vi "Edit Popup Menu.vi"(6 "User Menu States":bool[](array[boolean]), 7 "User Menu Items":string[](array[string]), 8 "error in (no error)":errorcluster, 10 "Menu Operation Cluster":T1(array[cluster]), 11 "Menu Ref In":refnum<k9>) -> (0 "error out":errorcluster, 3 "Menu Ref Out":refnum<k9>)   [LabVIEW 2017, in "2D Plot.lvclass"]
uses:
  <vilib>/Math Plots/2D Math Plots/2D Plot/2D Plot/2D Plot.lvclass
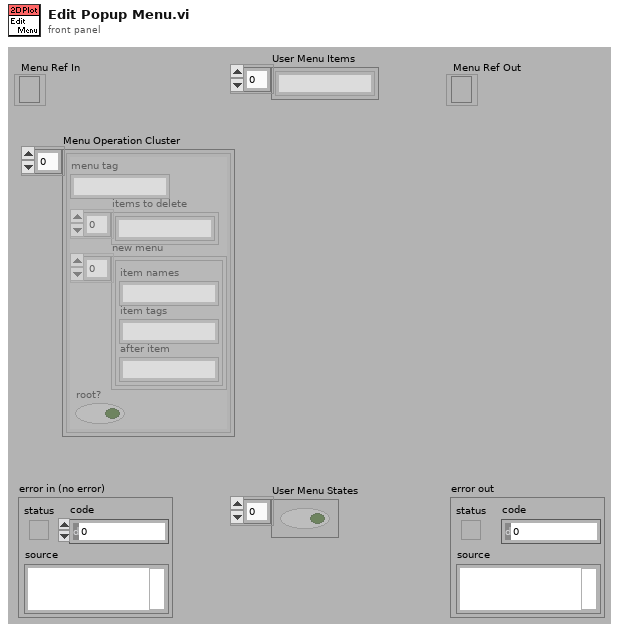
[diagram p1: front panel]
types:
  T1 = cluster{"menu tag":string, "items to delete":string[], "new menu":cluster{"item names":string, "item tags":string, "after item":string}[], "root?":bool}[]
  T2 = cluster{"item names":string, "item tags":string, "after item":string}[]
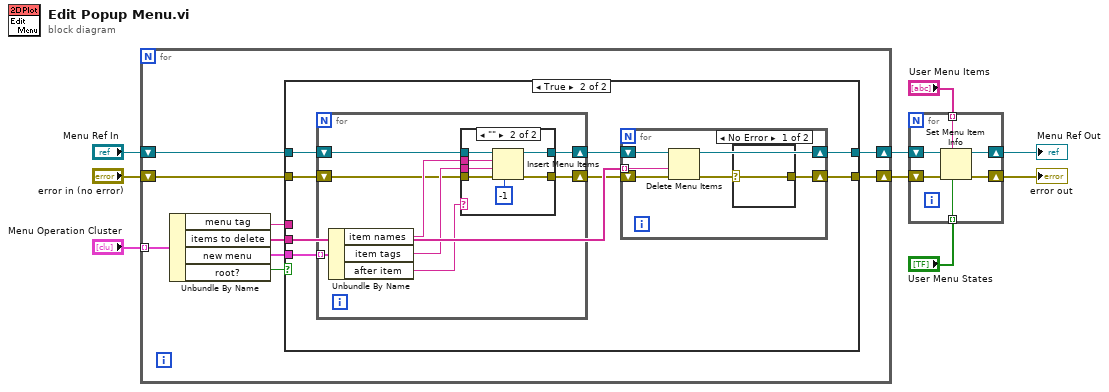
[diagram p0: block diagram]
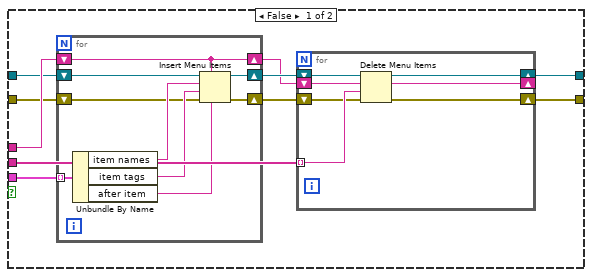
[diagram p2: hidden frame]
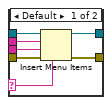
[diagram p3: hidden frame]
diagram:
  n1 = for {
    tunnel: "Menu Operation Cluster" -> [w18] mode=indexing
    shift-right: [w15] -> w6
    shift-left: "Menu Ref In" -> [w16]
    shift-right: [w11] -> w5
    shift-left: "error in (no error)" -> [w10]
    n2 = Unbundle By Name(w18) -> ("menu tag"=w14:string, "items to delete"=w13:string[], "new menu"=w12:T2, "root?"=w17:bool)
    n3 = case shown="True" w17 {
      tunnel: w16 -> [w20 w49]
      tunnel: w14 -> [w26 _]
      tunnel: w13 -> [w28 w50]
      tunnel: w12 -> [w27 w51]
      tunnel: [w21 w45] -> w15
      tunnel: [w22 w44] -> w11
      tunnel: w10 -> [w19 w48]
      frame False {
        n4 = for {
          shift-right: [w31] -> w24
          shift-left: w20 -> [w37]
          shift-right: [w36] -> w23
          shift-left: w26 -> [w36]
          tunnel: w27 -> [w35] mode=indexing
          shift-right: [w30] -> w25
          shift-left: w19 -> [w29]
          n5 = Unbundle By Name(w35) -> ("item names"=w34:string, "item tags"=w33:string, "after item"=w32:string)
          n6 = Insert Menu Items(4:w32, 5:w36, 6:w29, 7:w33, 8:w34, 9:w37) -> (0:w30:errorcluster, 3:w31:refnum<k9>)  [unwired: 1 out]
        }
        n7 = for {
          shift-right: [w42] -> w21
          shift-left: w24 -> [w43]
          shift-right: [w40] -> _
          shift-left: w23 -> [w40]
          tunnel: w28 -> [w41] mode=indexing
          shift-right: [w39] -> w22
          shift-left: w25 -> [w38]
          n8 = Delete Menu Items(6:w38, 7:w41, 8:w40, 9:w43) -> (0:w39:errorcluster, 3:w42:refnum<k9>)
        }
      }
      frame True {
        n9 = for {
          shift-right: [w59] -> w46
          shift-left: w49 -> [w58]
          tunnel: w51 -> [w57] mode=indexing
          shift-right: [w52] -> w47
          shift-left: w48 -> [w53]
          n10 = Unbundle By Name(w57) -> ("item names"=w56:string, "item tags"=w55:string, "after item"=w54:string)
          n11 = case shown="\"\"" w54 {
            selector: w54 -> [w64 _]
            tunnel: [w65 w73] -> w59
            tunnel: w58 -> [w66 w72]
            tunnel: w56 -> [w63 w71]
            tunnel: w55 -> [w62 w70]
            tunnel: w53 -> [w61 w68]
            tunnel: [w60 w67] -> w52
            frame Default {
              n12 = Insert Menu Items(4:w64, 6:w61, 7:w62, 8:w63, 9:w66) -> (0:w60:errorcluster, 3:w65:refnum<k9>)  [unwired: 2 out]
            }
            frame "" {
              n13 = Insert Menu Items(4:-1, 6:w68, 7:w70, 8:w71, 9:w72) -> (0:w67:errorcluster, 3:w73:refnum<k9>)  [unwired: 2 out]
            }
          }
        }
        n14 = for {
          shift-right: [w78] -> w45
          shift-left: w46 -> [w79]
          tunnel: w50 -> [w77] mode=indexing
          shift-right: [w74] -> w44
          shift-left: w47 -> [w76]
          n15 = Delete Menu Items(6:w76, 7:w77, 9:w79) -> (0:w75:errorcluster, 3:w78:refnum<k9>)  [unwired: 1 out]
          n16 = case shown="No Error" w75 {
            selector: w75 -> [w80 _]
            tunnel: [w80 _] -> w74
            frame No Error {
            }
            frame Error {
            }
          }
        }
      }
    }
  }
  n17 = for {
    shift-right: [w85] -> w1
    shift-left: w6 -> [w86]
    tunnel: "User Menu Items" -> [w84] mode=indexing
    tunnel: "User Menu States" -> [w83] mode=indexing
    shift-right: [w81] -> w9
    shift-left: w5 -> [w82]
    n18 = Set Menu Item Info(6:w83, 7:w84, 8:w82, 11:w86) -> (0:w81:errorcluster, 3:w85:refnum<k9>)  [unwired: 3 out]
  }
  "error out" <- w9
  "Menu Ref Out" <- w1
